vi "GetParam.vi"(8 "error in (no error)":errorcluster caption="entrée d'erreur (pas d'erreur)", 11 "OneHotEncoder.lvclass":refnum<class "OneHotEncoder.lvclass">) -> (0 "error out":errorcluster caption="sortie d'erreur", 2 "OneHotEncoder":T1={"drop"="None", "sparse"=TRUE, "dtype"="float", "handle_unknown"="error"}, 3 "OneHotEncoder.lvclass":refnum<class "OneHotEncoder.lvclass">)   [LabVIEW 2020, in "OneHotEncoder.lvclass"]
doc: "Get Parameters"
uses:
  OneHotEncoder.lvclass
  OneHotEncoder.lvclass/OneHotEncoder.ctl
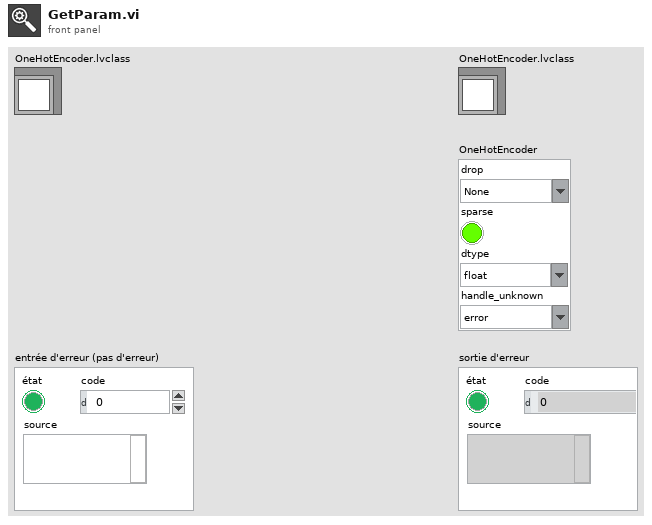
[diagram p1: front panel]
types:
  T1 = cluster{"drop":string, "sparse":bool, "dtype":string, "handle_unknown":string}
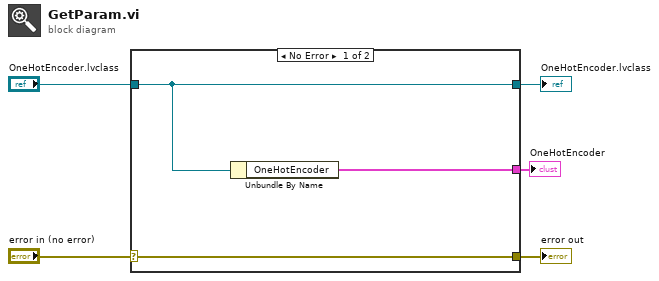
[diagram p0: block diagram]
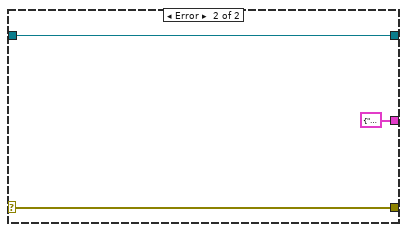
[diagram p2: hidden frame]
diagram:
  n1 = case shown="No Error" "error in (no error)" {
    selector: "error in (no error)" -> [w8 w10]
    tunnel: [w8 w10] -> w4
    tunnel: [w7 w11] -> w2
    tunnel: "OneHotEncoder.lvclass" -> [w7 w11]
    tunnel: [w6 T1 {"drop"="", "sparse"=FALSE, "dtype"="", "handle_unknown"=""} ("OneHotEncoder")] -> w1
    frame No Error {
      n2 = Unbundle By Name(w7) -> ("OneHotEncoder"=w6:T1)
    }
    frame Error {
    }
  }
  "error out" <- w4
  "OneHotEncoder.lvclass" <- w2
  "OneHotEncoder" <- w1
